vi "质控单元MB_api.vi"(6 "Slave ID":u8=1, 7 "STEP":enum16{"open", "read", "write", "close"}(ring)=enum."read", 8 "Error in":errorcluster caption="Error in (no error)", 9 "values":u16[](array[numeric]), 10 "quantity":u16, 11 "starting address":u16 format="%04xH") -> (0 "error out":errorcluster, 1 "MB session out":refnum<class "MB_Master.lvclass">, 2 "MB_TCP session":refnum<class "MB_Master_TCP.lvclass">, 3 "Registers":u16[](array[numeric]))   [LabVIEW 2016, in "质控单元.lvlib"]
uses:
  <vilib>/Plasmionique/MB Master/MB_Master/MB_Master.lvclass
  <vilib>/Plasmionique/MB Master/MB_Master_TCP/MB_Master_TCP.lvclass
  D:/Program Files (x86)/National Instruments/LabVIEW 2016/vi.lib/Plasmionique/MB Master/MB_Master/MB_Master.lvclass
  <vilib>/Plasmionique/MB Master/MB_Master_Serial/MB_Master_Serial.lvclass
  <vilib>/Plasmionique/MB Master/MB Master.lvlib
  <vilib>/Plasmionique/MB Master/MB_ADU_Serial/MB_ADU_Serial.lvclass
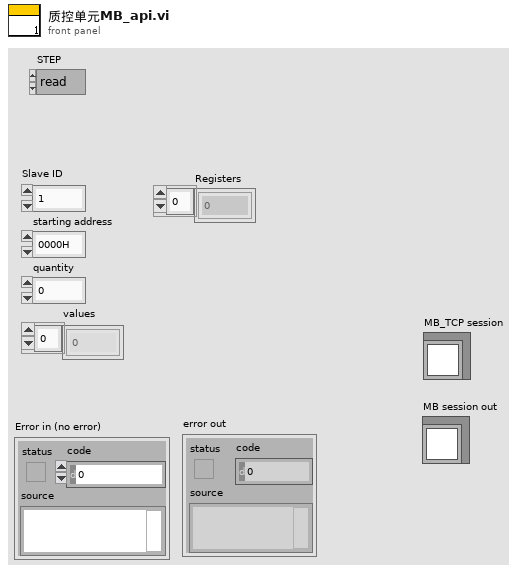
[diagram p1: front panel]
types:
  T1 = cluster{"baud rate (bps)":u32, "stop bits":u16, "parity":u16, "flow control":u16, "timeout":u32, "retries":i32}
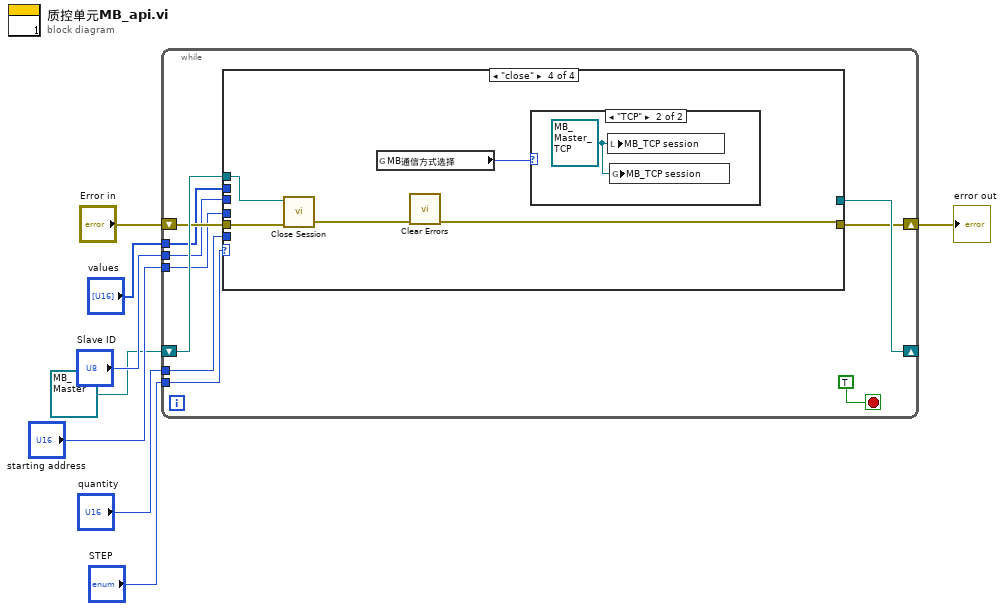
[diagram p0: block diagram]
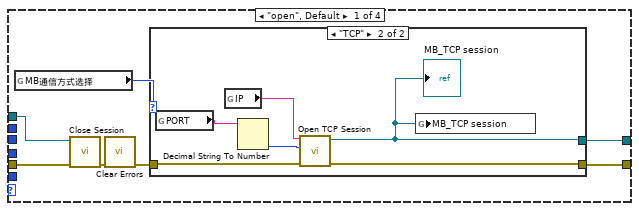
[diagram p2: hidden frame]
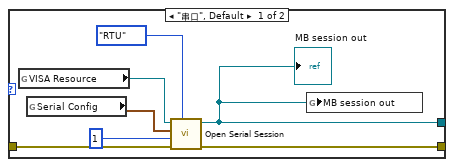
[diagram p3: hidden frame]
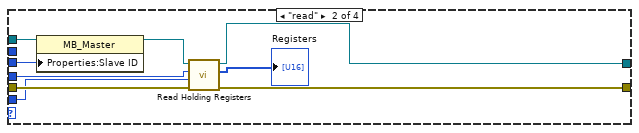
[diagram p4: hidden frame]
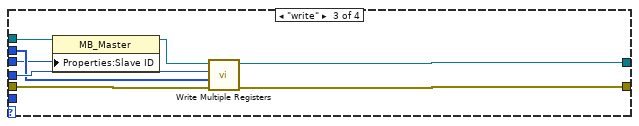
[diagram p5: hidden frame]
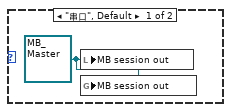
[diagram p6: hidden frame]
diagram:
  n1 = while {
    shift-right: [w12] -> _
    shift-left: refnum<class "MB_Master.lvclass"> refnum ("MB session out") -> [w18]
    shift-right: [w11] -> w7
    shift-left: "Error in" -> [w17]
    tunnel: "Slave ID" -> [w16]
    tunnel: "starting address" -> [w15]
    tunnel: "quantity" -> [w14]
    tunnel: "STEP" -> [w13]
    tunnel: "values" -> [w10]
    stop <- TRUE stop-if-true
    n2 = case shown="\"close\"" w13 {
      tunnel: w18 -> [w23 w40 w50 w59]
      tunnel: w17 -> [w22 w47 w55 w60]
      tunnel: [w24 w46 w53 _] -> w12
      tunnel: [w25 w45 w54 w57] -> w11
      tunnel: w16 -> [_ w43 w49 _]
      tunnel: w15 -> [_ w42 w52 _]
      tunnel: w14 -> [_ w41 _ _]
      tunnel: w10 -> [_ _ w51 _]
      frame "open", Default {
        n3 = global read "断电保存全局.vi" "MB通信方式选择"() -> (w19:enum16{"串口", "TCP"})
        n4 = call-dynamic "Close Session.vi"("error in (no error)"=w22, "MB session in"=w23) -> ("error out"=w21:errorcluster)  [unwired: 9 in]
        n5 = call <vilib>:"Clear Errors.vi"("error in (no error)"=w21) -> ("error out"=w20:errorcluster)  [unwired: 5 in, 1 out]
        n6 = case shown="\"TCP\"" w19 {
          tunnel: [w31 w35] -> w25
          tunnel: [w27 w33] -> w24
          tunnel: w20 -> [w28 w34]
          frame "串口", Default {
            n7 = global read "断电保存全局.vi" "VISA Resource"() -> (w30:refnum<visa-resource-name>)
            n8 = global read "断电保存全局.vi" "Serial Config"() -> (w29:T1)
            n9 = call <vilib>:"Open Serial Session.vi"("Mode (RTU)"=enum16{"RTU", "ASCII"}."RTU", "Error in"=w28, "Slave ID"=u8 1, "Serial Config"=w29, "VISA Resource"=w30) -> ("Error out"=w31:errorcluster, "MB_Serial session"=w27:refnum<class "MB_Master_Serial.lvclass">)  [unwired: 5 in]
            "MB session out" <- w27
            n10 = global write "断电保存全局.vi" "MB session out"(w27) -> ()
          }
          frame "TCP" {
            n11 = global read "断电保存全局.vi" "PORT"() -> (w37:string)
            n12 = global read "断电保存全局.vi" "IP"() -> (w36:string)
            n13 = Decimal String To Number(string=w37) -> (number=w38:i32)  [unwired: 2 in, 1 out]
            n14 = call <vilib>:"Open TCP Session.vi"("error in (no error)"=w34, "Port (502)"=w38, "IP Address"=w36) -> ("error out"=w35:errorcluster, "MB_TCP session"=w33:refnum<class "MB_Master_TCP.lvclass">)  [unwired: 7 in]
            "MB_TCP session" <- w33
            n15 = global write "断电保存全局.vi" "MB_TCP session"(w33) -> ()
          }
        }
      }
      frame "read" {
        n16 = property class="MB_Master"(reference=w40, "Properties:Slave ID"=w43) -> (reference out=w39:refnum<class "MB_Master.lvclass">)  [unwired: 1 in, 1 out]
        n17 = call <vilib>:"Read Holding Registers.vi"("error in (no error)"=w47, "quantity"=w41, "starting address"=w42, "MB session in"=w39) -> ("error out"=w45:errorcluster, "Registers"=→"Registers":u16[], "MB session out"=w46:refnum<class "MB_Master.lvclass">)  [unwired: 5 in]
      }
      frame "write" {
        n18 = property class="MB_Master"(reference=w50, "Properties:Slave ID"=w49) -> (reference out=w48:refnum<class "MB_Master.lvclass">)  [unwired: 1 in, 1 out]
        n19 = call <vilib>:"Write Multiple Registers.vi"("error in (no error)"=w55, "values"=w51, "starting address"=w52, "MB session in"=w48) -> ("error out"=w54:errorcluster, "MB session out"=w53:refnum<class "MB_Master.lvclass">)  [unwired: 6 in]
      }
      frame "close" {
        n20 = call-dynamic "Close Session.vi"("error in (no error)"=w60, "MB session in"=w59) -> ("error out"=w58:errorcluster)  [unwired: 9 in]
        n21 = global read "断电保存全局.vi" "MB通信方式选择"() -> (w56:enum16{"串口", "TCP"})
        n22 = call <vilib>:"Clear Errors.vi"("error in (no error)"=w58) -> ("error out"=w57:errorcluster)  [unwired: 5 in, 1 out]
        n23 = case shown="\"TCP\"" w56 {
          frame "串口", Default {
            w61 = refnum<class "MB_Master.lvclass"> refnum ("MB session out")
            n24 = local write "MB session out"(w61) -> ()
            n25 = global write "断电保存全局.vi" "MB session out"(w61) -> ()
          }
          frame "TCP" {
            w62 = refnum<class "MB_Master_TCP.lvclass"> refnum ("MB_TCP session")
            n26 = local write "MB_TCP session"(w62) -> ()
            n27 = global write "断电保存全局.vi" "MB_TCP session"(w62) -> ()
          }
        }
      }
    }
  }
  "error out" <- w7
